vi "PI_GCS3_Sample_Application_DataRecorder.vi"() -> ()   [LabVIEW 2020]
doc: "This VI demonstrates how to use the PI GCS3 data recorder functionality. The diagram shows how to combine the driver VIs for these tasks.\n\nWarning: Before running this VI, modify the interface settings on the block diagram to reflect your configuration. The predefined settings provided with the VI probably do not match your system.\n\nCompatibility: This sample requires a PI GCS 3.0 controller."
uses:
  Low Level/Special command.llb/RecorderTriggerConfiguration.ctl
  Low Level/Special command.llb/RecorderTraceConfiguration.ctl
  Low Level/Special command.llb/ModeOfOperation.ctl
  Low Level/Communication.llb/Interface Settings.ctl
panel:
  out "Recorded data points":i32[](array[numeric])
  out "Position Error of AXIS_1":waveform(dbl)(graph)
  out "Generated Position of AXIS_1":waveform(dbl)(graph)
  out "Real Position of AXIS_1":waveform(dbl)(graph)
  out "Conn. Axes":string[](array[string])
  out "Identification":string
  out "error out":errorcluster
  in  "error in (no error)":errorcluster
  # "This VI demonstrates how to use the PI GCS3 data recorder functionality.\nThe diagram shows how to combine the driver VIs for these tasks. \n\nWarning: Before running this VI, modify the interface settings on the block diagram to reflect your configuration.\n                 The predefined settings provided with the VI probably do not match your system.\n\nCompatibility: This sample requires a PI GCS 3.0 controller."
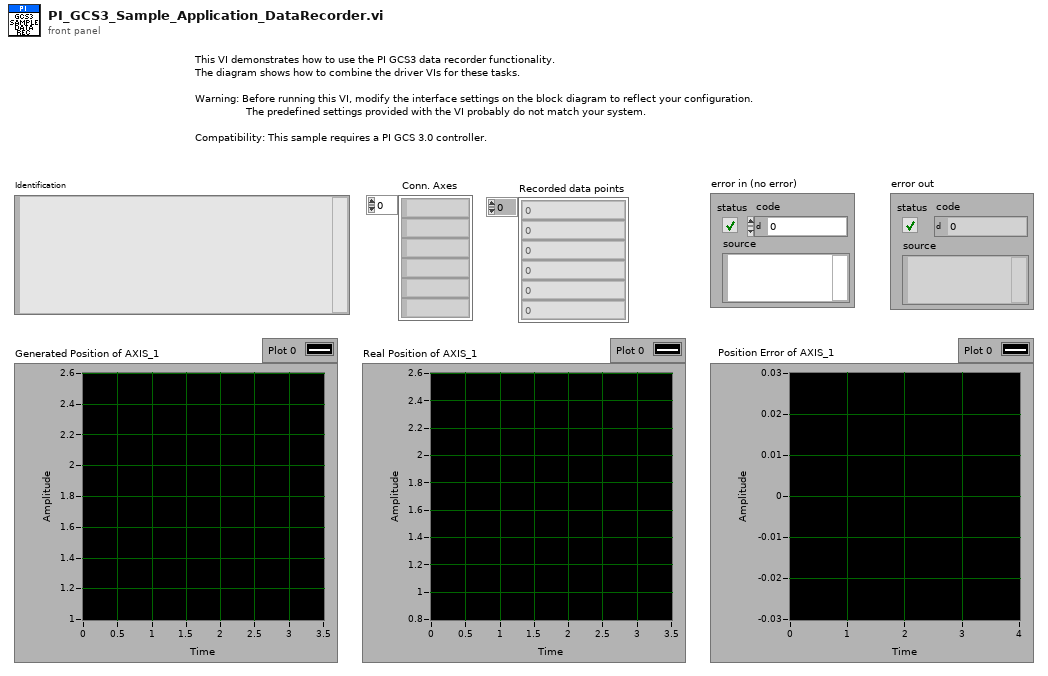
[diagram p1: front panel]
types:
  T1 = typedef "Interface Settings.ctl" = cluster{"Interface":u16, "Timeout":u32, "RS232 settings":cluster{"Portnumber":u8, "Baudrate":u16}, "TCP/IP settings":cluster{"Host address/name":string, "Port":i32, "Board":i32, "TCP/IP Search?":bool}, "USB settings":cluster{"S/N":string, "USB Search?":bool}, "DaisyChain settings":cluster{"Register DC":bool, "DaisyChain Search?":bool, "Device ID":i32}, "DLL for Device":u16}
  T2 = typedef "ModeOfOperation.ctl" = enum16{"Open", "Open-Loop Position", "Closed-Loop Position", "Open-Loop Velocity", "Closed-Loop Velocity", "Open-Loop Force", "Closed-Loop Force", "Step Operation"}
  T3 = typedef "RecorderTraceConfiguration.ctl" = cluster{"RecorderID":string, "TraceID":i32, "Container Unit":string, "Function Unit":string, "ParameterID":i32}
  T4 = typedef "RecorderTriggerConfiguration.ctl" = cluster{"RecorderID":string, "RecorderTrigger":string, "AxisID":string, "Recurring":string}
  T5 = typedef "GCSArray_header.ctl" = cluster{"Identifier":string, "Version":i32, "Remark":string, "Dimension":i32, "Type":enum16{"Matrix", "Table"}, "Separator":u8, "NData":i32, "NData%":i32[], "Name%":string[], "Start%":dbl[], "End%":dbl[], "Delta%":dbl[], "SampleTime":dbl, "TransmittedUnit%":string[], "DisplayedUnit%":string[], "RatioNominator%":dbl[], "RatioDenominator%":dbl[]}
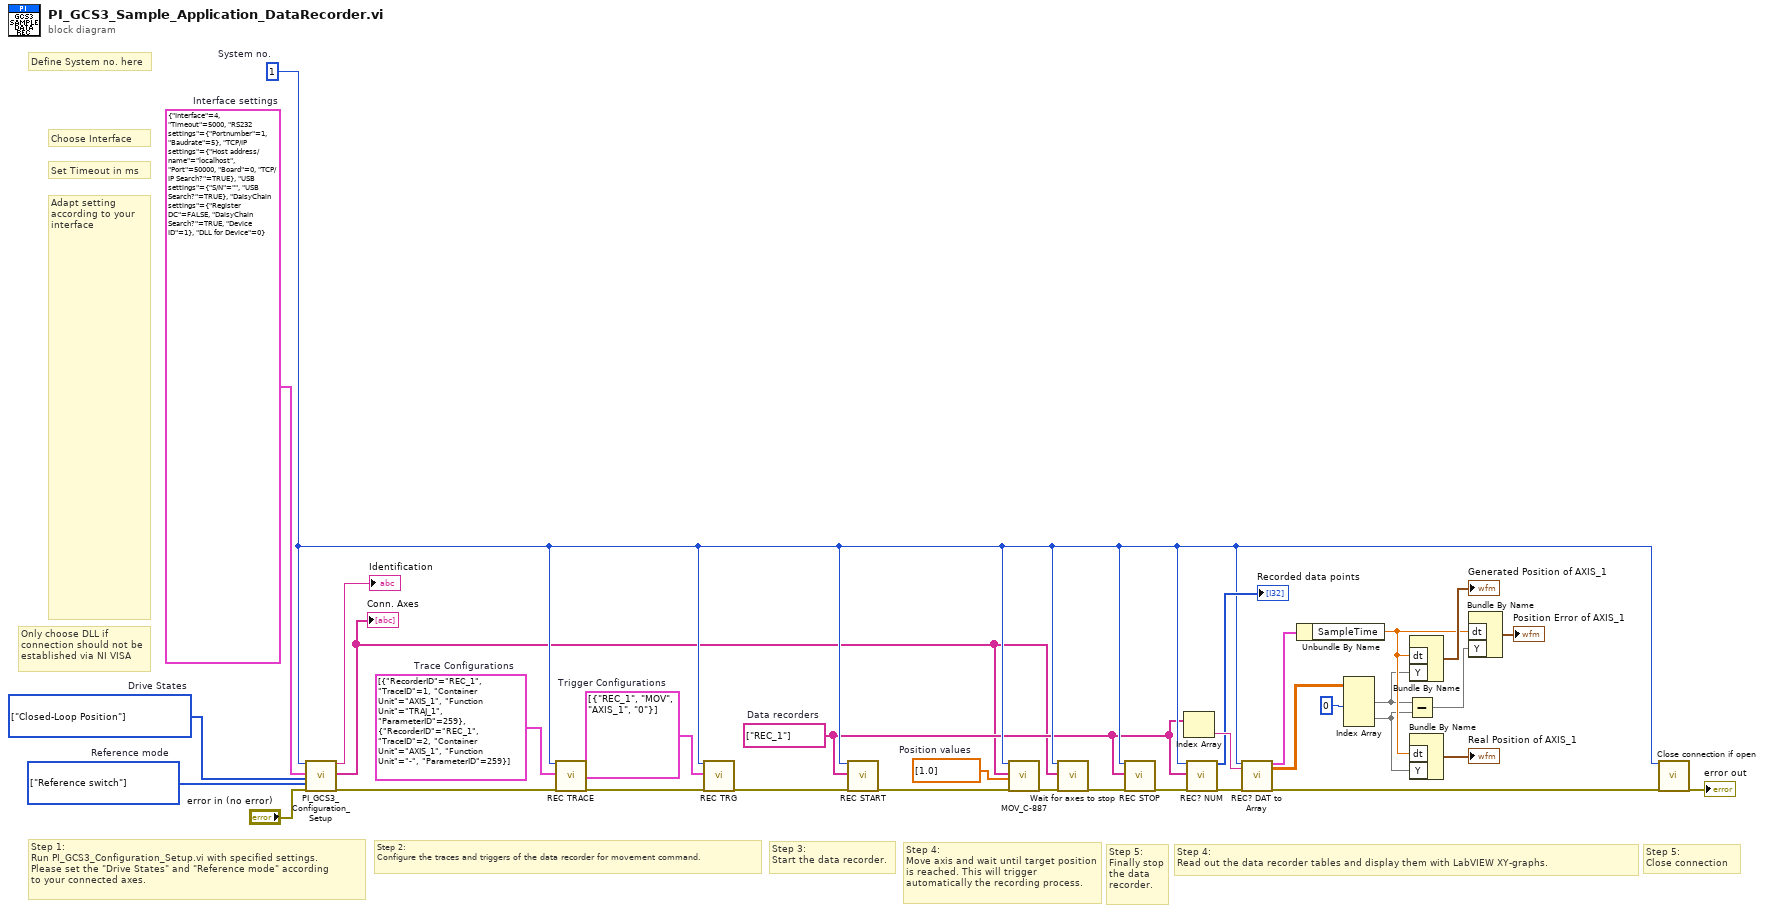
[diagram p0: block diagram]
diagram:
  w1 = T1 {"Interface"=4, "Timeout"=5000, "RS232 settings"={"Portnumber"=1, "Baudrate"=5}, "TCP/IP settings"={"Host address/name"="localhost", "Port"=50000, "Board"=0, "TCP/IP Search?"=TRUE}, "USB settings"={"S/N"="", "USB Search?"=TRUE}, "DaisyChain settings"={"Register DC"=FALSE, "DaisyChain Search?"=TRUE, "Device ID"=1}, "DLL for Device"=0}  # Interface settings
  w8 = enum16{"Do not reference", "Reference switch"}[] [enum."Reference switch"] items=["Do not reference", "Reference switch"]  # Reference mode
  w10 = T2[] [enum."Closed-Loop Position"] items=["Open", "Open-Loop Position", "Closed-Loop Position", "Open-Loop Velocity", "Closed-Loop Velocity", "Open-Loop Force", "Closed-Loop Force", "Step Operation"]  # Drive States
  w4 = 1  # System no.
  w27 = T3[] [{"RecorderID"="REC_1", "TraceID"=1, "Container Unit"="AXIS_1", "Function Unit"="TRAJ_1", "ParameterID"=259}, {"RecorderID"="REC_1", "TraceID"=2, "Container Unit"="AXIS_1", "Function Unit"="-", "ParameterID"=259}]  # Trace Configurations
  w32 = dbl[] [1.0]  # Position values
  w33 = T4[] [{"RecorderID"="REC_1", "RecorderTrigger"="MOV", "AxisID"="AXIS_1", "Recurring"="0"}]  # Trigger Configurations
  w3 = string[] ["REC_1"]  # Data recorders
  # "Define System no. here"
  # "Adapt setting according to your interface"
  # "Set Timeout in ms"
  # "Choose Interface"
  # "Only choose DLL if connection should not be established via NI VISA"
  # "Step 5:\nFinally stop\nthe data recorder."
  # "Step 4:\nMove axis and wait until target position is reached. This will trigger automatically the recording process."
  # "Step 4:\nRead out the data recorder tables and display them with LabVIEW XY-graphs."
  # "Step 3:\nStart the data recorder."
  # "Step 2:\nConfigure the traces and triggers of the data recorder for movement command."
  # "Step 5:\nClose connection"
  # "Step 1:\nRun PI_GCS3_Configuration_Setup.vi with specified settings.\nPlease set the \"Drive States\" and \"Reference mode\" according\nto your connected axes."
  n1 = call "PI_GCS3_Configuration_Setup.vi"("System no."=w4, "Interface settings"=w1, "Mode of operation"=w10, "Reference mode"=w8, "error in"="error in (no error)") -> ("Identification"=→"Identification":string, "Conn. axis"=w2:string[], "error out"=w9:errorcluster)  [unwired: 9 in, 3 out]
  "Conn. Axes" <- w2
  n2 = call "REC TRACE.vi"("System no."=w4, "List of Data Recorder Trace Configurations"=w27, "error in"=w9) -> ("error out"=w28:errorcluster)  [unwired: 16 in]
  n3 = call "REC TRG.vi"("System no."=w4, "List of Data Recorder Trigger Configurations"=w33, "error in"=w28) -> ("error out"=w30:errorcluster)  [unwired: 16 in]
  n4 = call "REC START.vi"("System no."=w4, "RecorderIDs"=w3, "error in"=w30) -> ("error out"=w29:errorcluster)  [unwired: 16 in]
  n5 = call "MOV_C-887.vi"("System no."=w4, "Axes to move"=w2, "Position values"=w32, "error in"=w29) -> ("error out"=w31:errorcluster)  [unwired: 15 in]
  n6 = call "Wait for axes to stop.vi"("System no."=w4, "Axes to wait for"=w2, "error in"=w31) -> ("error out"=w25:errorcluster)  [unwired: 15 in, 1 out]
  n7 = call "REC STOP.vi"("System no."=w4, "RecorderIDs"=w3, "error in"=w25) -> ("error out"=w14:errorcluster)  [unwired: 16 in]
  n8 = Index Array(array=w3) -> (element=w26:string)  [unwired: 1 in]
  n9 = call "REC? NUM.vi"("System no."=w4, "RecorderIDs to query"=w3, "error in"=w14) -> ("Number of recorded data points"=→"Recorded data points":i32[], "error out"=w13:errorcluster)  [unwired: 15 in]
  n10 = call "REC? DAT to Array.vi"("System no."=w4, "RecorderID"=w26, "error in"=w13) -> ("GCSArray Header"=w23:T5, "GCSArray data"=w24:dbl[][], "error out"=w6:errorcluster)  [unwired: 14 in]
  n11 = Unbundle By Name(w23) -> ("SampleTime"=w19:dbl)
  n12 = Index Array(array=w24, index (col) #1=0 ("disabled index (col)")) -> (element #1=w17:dbl[], element #2=w16:dbl[])  [unwired: 3 in]
  n13 = Subtract(x=w17, y=w16) -> (x-y=w15:dbl[])
  n14 = Bundle By Name("dt"=w19, "Y"=w17) -> (→"Generated Position of AXIS_1":waveform(dbl))  [unwired: 1 in]
  n15 = Bundle By Name("dt"=w19, "Y"=w16) -> (→"Real Position of AXIS_1":waveform(dbl))  [unwired: 1 in]
  n16 = Bundle By Name("dt"=w19, "Y"=w15) -> (→"Position Error of AXIS_1":waveform(dbl))  [unwired: 1 in]
  n17 = call "Close connection if open.vi"("System no."=w4, "error in"=w6) -> ("error out"=→"error out":errorcluster)  [unwired: 16 in, 1 out]
